vi "Get_link_info.vi"(5 "VI Name":string) -> (0 "badServer":bool, 1 "Application reference":refnum<vi>, 2 "Path name":path, 3 "Server IP & Port":string, 4 "Local Call?":bool)   [LabVIEW 2020]
uses:
  Anemometry/Anemometry Sub Vis/Controls/Serveds.ctl
  Anemometry/Anemometry Sub Vis/Controls/App_Global.ctl
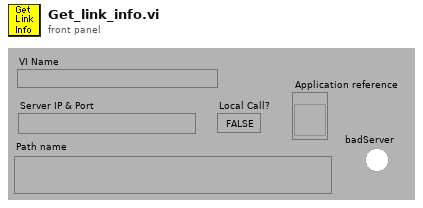
[diagram p1: front panel]
types:
  T1 = typedef "App_Global.ctl" = enum16{"Read Global", "Write to Global", "Initialise Array"}
  T2 = typedef "Serveds.ctl" = enum16{"Read Global", "Load Global From File"}
  T3 = typedef "App_Ref_Cluster.ctl" = cluster{"Server IP & Port No":string, "Application reference":refnum<vi>}
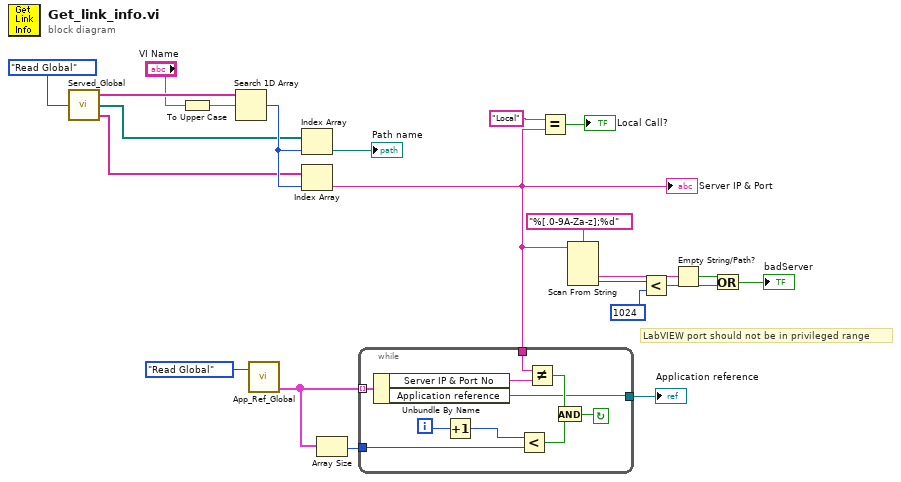
[diagram p0: block diagram]
diagram:
  # "LabVIEW port should not be in privileged range"
  n1 = call "Served_Global.vi"("Mode"=Serveds."Read Global") -> ("Served VI Name"=w19:string[], "Served VI Path"=w17:path[], "Served IP Number & Port No"=w18:string[])
  n2 = To Upper Case(1:"VI Name") -> (0:w13:string)
  n3 = Search 1D Array(1D array=w19, element=w13) -> (index of element=w22:i32)  [unwired: 1 out]
  n4 = call "App_Ref_Global.vi"("Mode"=App_Global."Read Global") -> ("Output Array"=w11:T3[])  [unwired: 1 in, 1 out]
  n5 = Index Array(array=w17, index=w22) -> (element=→"Path name":path)
  n6 = Index Array(array=w18, index=w22) -> (element=w7:string)
  "Server IP & Port" <- w7
  n7 = Array Size(array=w11) -> (size(s)=w10:i32)
  n8 = while {
    tunnel: [w23] -> w9
    tunnel: w10 -> [w28]
    tunnel: w7 -> [w30]
    tunnel: w11 -> [w32] mode=indexing
    i -> [w29]
    stop <- w24 continue-if-true
    n9 = Unbundle By Name(w32) -> ("Server IP & Port No"=w31:string, "Application reference"=w23:refnum<vi>)
    n10 = Increment(x=w29) -> (x+1=w27:i32)
    n11 = Less?(x=w27, y=w28) -> (x < y?=w26:bool)
    n12 = Not Equal?(x=w30, y=w31) -> (x != y?=w25:bool)
    n13 = And(x=w25, y=w26) -> (x .and. y?=w24:bool)
  }
  "Application reference" <- w9
  n14 = Equal?(x="Local" ("t"), y=w7) -> (x = y?=→"Local Call?":bool)
  n15 = Scan From String(format string="%[.0-9A-Za-z];%d", input string=w7) -> (output 1=w4:string, output 2=w5:i32)  [unwired: 4 in, 3 out]
  n16 = Less?(x=w5, y=1024) -> (x < y?=w2:bool)
  n17 = Empty String/Path?(string/path=w4) -> (empty?=w3:bool)
  n18 = Or(x=w3, y=w2) -> (x .or. y?=→"badServer":bool)
